vi "Graph mit Bemerkung.vi"(0 "Context (Eingang)":refnum<class "Context.lvclass">, 1 "Table Configuration":T4={"Table Settings"={"Number of Columns"=1, "Width (%)"=100.0, "Relative Column Widths (%)"=[100.0], "Horizontal Align"=0, "Header Rows"=0}, "Cell Defaults"={"Background Color"=16777215, "Horizontal Align"=0, "Vertical Align"=1, "Minimum Height"=0.0, "Fixed Height"=0.0, "Padding"={"Left"=0.0, "Top"=0.0, "Right"=0.0, "Bottom"=0.0}}, "Borders"={"Left"={"Enabled"=FALSE, "Width"=1.0, "Color"=0}, "Top"={"Enabled"=FALSE, "Width"=1.0, "Color"=0}, "Right"={"Enabled"=FALSE, "Width"=1.0, "Color"=0}, "Bottom"={"Enabled"=FALSE, "Width"=1.0, "Color"=0}, "Middle Horizontal"={"Enabled"=FALSE, "Width"=0.5, "Color"=0}, "Middle Vertical"={"Enabled"=FALSE, "Width"=0.5, "Color"=0}}} {"Cell Defaults"."Vertical Align" items=["Bottom", "Middle", "Top"]; "Cell Defaults"."Horizontal Align" items=["Center", "Justified", "JustifiedAll", "Left", "Right"]; "Table Settings"."Horizontal Align" items=["Center"=0, "Left"=3, "Right"=4]}, 2 "Cell Configuration":T1={"Cell Defaults"={"Background Color"=16777215, "Horizontal Align"=0, "Vertical Align"=1, "Minimum Height"=0.0, "Fixed Height"=0.0, "Padding"={"Left"=0.0, "Top"=0.0, "Right"=0.0, "Bottom"=0.0}}, "Borders"={"Left"={"Enabled"=FALSE, "Width"=1.0, "Color"=0}, "Top"={"Enabled"=FALSE, "Width"=1.0, "Color"=0}, "Right"={"Enabled"=FALSE, "Width"=1.0, "Color"=0}, "Bottom"={"Enabled"=FALSE, "Width"=1.0, "Color"=0}}, "Column Span"=0} {"Cell Defaults"."Vertical Align" items=["Bottom", "Middle", "Top"]; "Cell Defaults"."Horizontal Align" items=["Center", "Justified", "JustifiedAll", "Left", "Right"]}, 5 "Graph":T6={"GraphCtl Refnum"=refnum, "Wrap Text (F:No)"=FALSE, "Hide Grid (F:No)"=FALSE, "Scale (100%)"=100.0, "Align (Left)"=0, "PositionBemerkung"=enum."before", "PageBreak"=enum."before"} {"Align (Left)" items=["Center", "Justified", "Justified All", "Left", "Right"]}, 7 "Bemerkung Index (Eingang)":i32, 11 "Fehler (Eingang, kein Fehler)":errorcluster, 12 "Bemerkungen":T10[](array[typedef]) {"Align (Left)" items=["Center", "Justified", "Justified All", "Left", "Right"]}) -> (4 "Context (Ausgang)":refnum<class "Context.lvclass">, 8 "Bemerkung Index (Ausgang)":i32, 15 "Fehler (Ausgang)":errorcluster)   [LabVIEW 2020, in "PDF Interface.lvlib" / "PDF Interface Helper.lvlib"]
uses:
  PDF Interface Helper.lvlib
  PDFBemerkung.ctl
  <vilib>/Simplicity AI/SAI_PDF_API/Classes/Context/Controls/SAI_PDF_Text Align.ctl
  <vilib>/Simplicity AI/SAI_PDF_API/Classes/Context/Controls/SAI_PDF_Font.ctl
  <vilib>/Simplicity AI/SAI_PDF_API/Classes/Context/Controls/SAI_PDF_Font Encoding.ctl
  <vilib>/Simplicity AI/SAI_PDF_API/Classes/Context/Context.lvclass
  PDFGraph.ctl
  PDFCommentPosition.ctl
  PDFPageBreak.ctl
  <vilib>/Simplicity AI/SAI_PDF_API/Classes/Table Builder/Controls/SAI_PDF_Table Configuration.ctl
  <vilib>/Simplicity AI/SAI_PDF_API/Classes/Table Builder/Controls/SAI_PDF_Table Horizontal Align.ctl
  <vilib>/Simplicity AI/SAI_PDF_API/Classes/Table Builder/Controls/SAI_PDF_Default Cell Format.ctl
  <vilib>/Simplicity AI/SAI_PDF_API/Classes/Table Builder/Controls/SAI_PDF_BorderLine.ctl
  <vilib>/Simplicity AI/SAI_PDF_API/Classes/Table Builder/Controls/SAI_PDF_Cell Configuration.ctl
  <vilib>/Simplicity AI/SAI_PDF_API/Classes/Table Builder/Table Builder.lvclass
panel:
  # "(Cp1252)"
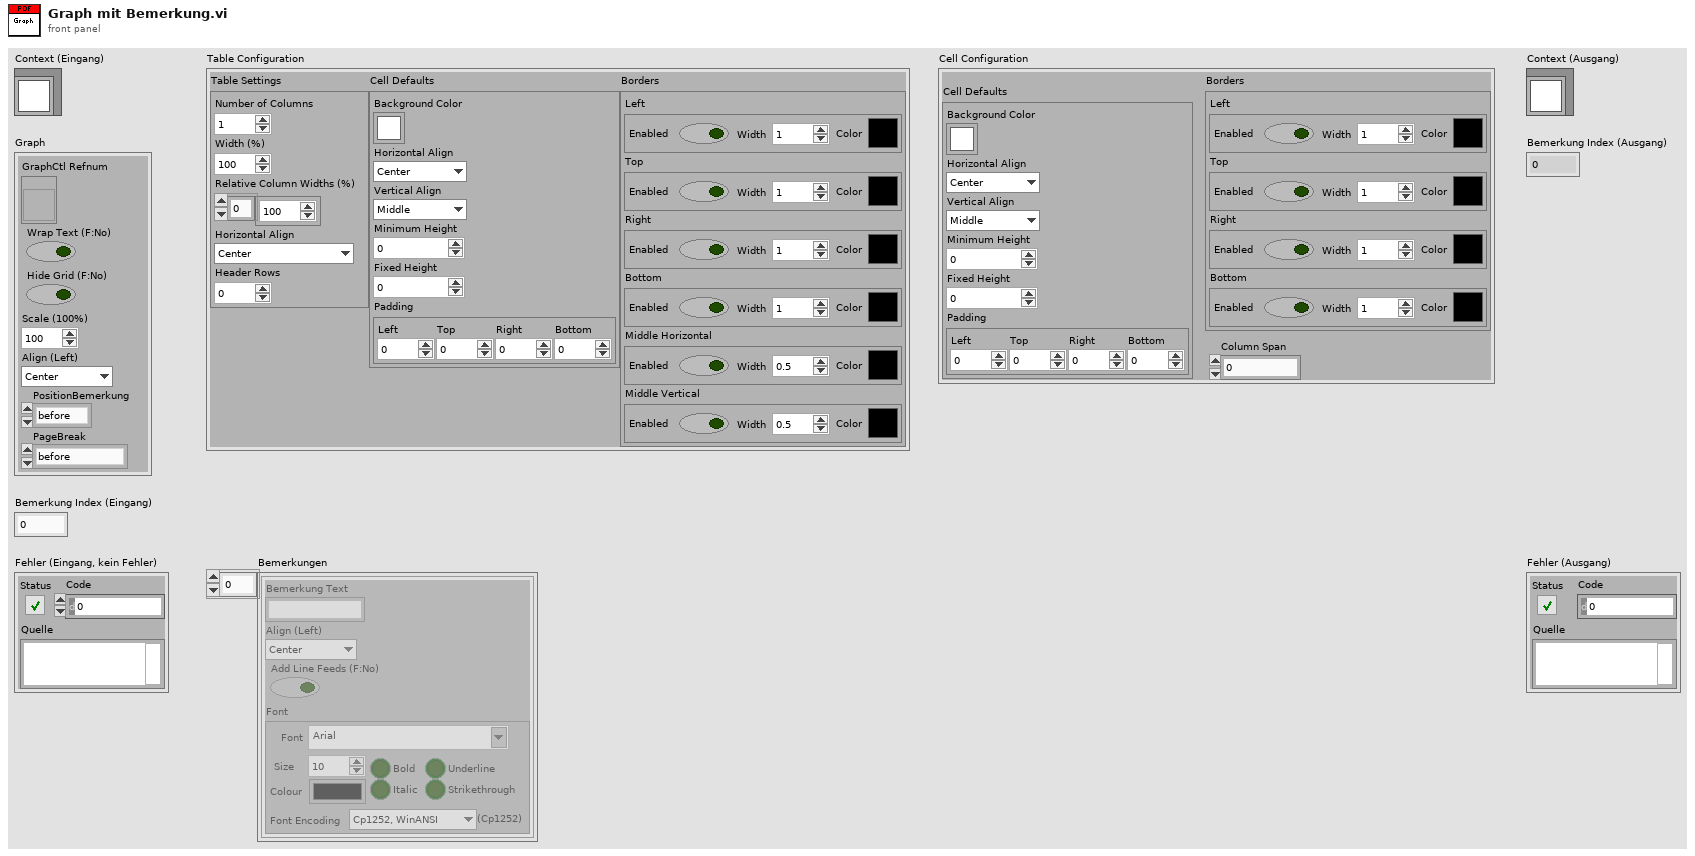
[diagram p1: front panel]
types:
  T1 = typedef "SAI_PDF_Toolkit.lvlib/Table Builder.lvclass/SAI_PDF_Cell Configuration.ctl" = cluster{"Cell Defaults":T2, "Borders":cluster{"Left":T3, "Top":T3, "Right":T3, "Bottom":T3}, "Column Span":i32}
  T2 = typedef "SAI_PDF_Toolkit.lvlib/Table Builder.lvclass/SAI_PDF_Default Cell Format.ctl" = cluster{"Background Color":u32, "Horizontal Align":i32, "Vertical Align":i32, "Minimum Height":sgl, "Fixed Height":sgl, "Padding":cluster{"Left":sgl, "Top":sgl, "Right":sgl, "Bottom":sgl}}
  T3 = typedef "SAI_PDF_Toolkit.lvlib/Table Builder.lvclass/SAI_PDF_BorderLine.ctl" = cluster{"Enabled":bool, "Width":sgl, "Color":u32}
  T4 = typedef "SAI_PDF_Toolkit.lvlib/Table Builder.lvclass/SAI_PDF_Table Configuration.ctl" = cluster{"Table Settings":cluster{"Number of Columns":i32, "Width (%)":sgl, "Relative Column Widths (%)":sgl[], "Horizontal Align":T5, "Header Rows":i32}, "Cell Defaults":T2, "Borders":cluster{"Left":T3, "Top":T3, "Right":T3, "Bottom":T3, "Middle Horizontal":T3, "Middle Vertical":T3}}
  T5 = typedef "SAI_PDF_Toolkit.lvlib/Table Builder.lvclass/SAI_PDF_Table Horizontal Align.ctl" = i32
  T6 = typedef "PDF Interface.lvlib/PDF Interface Helper.lvlib/PDFGraph.ctl" = cluster{"GraphCtl Refnum":refnum<vi>, "Wrap Text (F:No)":bool, "Hide Grid (F:No)":bool, "Scale (100%)":sgl, "Align (Left)":T7, "PositionBemerkung":T8, "PageBreak":T9}
  T7 = typedef "SAI_PDF_Toolkit.lvlib/Context.lvclass/SAI_PDF_Text Align.ctl" = i32
  T8 = typedef "PDF Interface.lvlib/PDF Interface Helper.lvlib/PDFCommentPosition.ctl" = enum16{"before", "after"}
  T9 = typedef "PDF Interface.lvlib/PDF Interface Helper.lvlib/PDFPageBreak.ctl" = enum16{"none", "before", "after", "after comment"}
  T10 = typedef "PDF Interface.lvlib/PDF Interface Helper.lvlib/PDFBemerkung.ctl" = cluster{"Bemerkung Text":string, "Align (Left)":T7, "Add Line Feeds (F:No)":bool, "Font":T11}
  T11 = typedef "SAI_PDF_Toolkit.lvlib/Context.lvclass/SAI_PDF_Font.ctl" = cluster{"Font":string, "Size":i32, "Colour":u32, "Bold":bool, "Italic":bool, "Underline":bool, "Strikethrough":bool, "Font Encoding":T12}
  T12 = typedef "SAI_PDF_Toolkit.lvlib/Context.lvclass/SAI_PDF_Font Encoding.ctl" = enum16{"Cp1252, WinANSI", "IdentityH", "IdentityV", "Cp1250", "Cp1257", "MacRoman"}
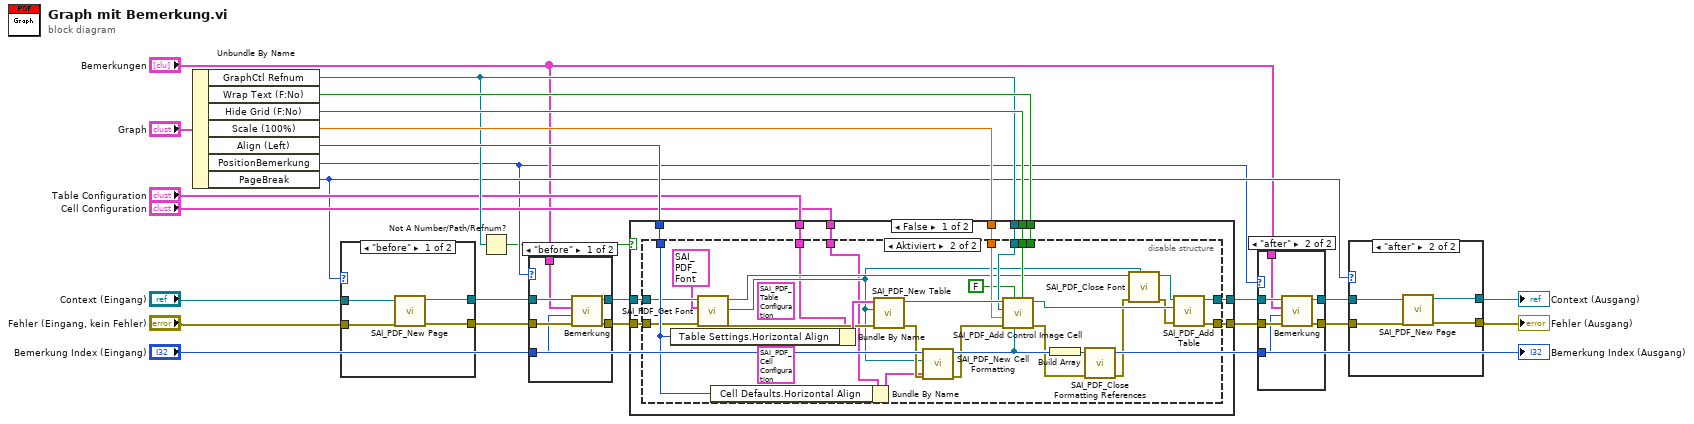
[diagram p0: block diagram]
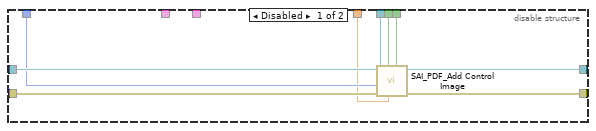
[diagram p2: hidden frame]
diagram:
  n1 = Unbundle By Name("Graph") -> ("GraphCtl Refnum"=w19:refnum<vi>, "Wrap Text (F:No)"=w23:bool, "Hide Grid (F:No)"=w22:bool, "Scale (100%)"=w21:sgl, "Align (Left)"=w20:T7, "PositionBemerkung"=w6:T8, "PageBreak"=w8:T9)
  n2 = case shown="\"before\"" w8 {
    tunnel: "Context (Eingang)" -> [w29 w31]
    tunnel: [w28 w31] -> w16
    tunnel: "Fehler (Eingang, kein Fehler)" -> [w27 w30]
    tunnel: [w26 w30] -> w15
    frame "before" {
      n3 = call <vilib>:"SAI_PDF_New Page.vi"("error in"=w27, "Context In"=w29) -> ("error out"=w26:errorcluster, "Context Out"=w28:refnum<class "Context.lvclass">)  [unwired: 8 in]
    }
    frame "after", Default {
    }
  }
  n4 = Not A Number/Path/Refnum?(number/path/refnum=w19) -> (NaN/Path/Refnum?=w1:bool)
  n5 = case shown="\"before\"" w6 {
    tunnel: w16 -> [w37 w39]
    tunnel: [w36 w39] -> w3
    tunnel: w15 -> [w35 w38]
    tunnel: [w34 w38] -> w2
    tunnel: "Bemerkung Index (Eingang)" -> [w33 _]
    tunnel: "Bemerkungen" -> [w32 _]
    frame "before" {
      n6 = call "Bemerkung.vi"("Fehler (Eingang, kein Fehler)"=w35, "Index"=w33, "Bemerkung"=w32, "Context (Eingang)"=w37) -> ("Fehler (Ausgang)"=w34:errorcluster, "Context (Ausgang)"=w36:refnum<class "Context.lvclass">)  [unwired: 6 in]
    }
    frame "after", Default {
    }
  }
  n7 = case shown="False" w1 {
    tunnel: [w50 w88] -> w5
    tunnel: [w49 w87] -> w4
    tunnel: w19 -> [w48 _]
    tunnel: w23 -> [w47 _]
    tunnel: w22 -> [w46 _]
    tunnel: w20 -> [w45 _]
    tunnel: w21 -> [w44 _]
    tunnel: "Table Configuration" -> [w43 _]
    tunnel: "Cell Configuration" -> [w42 _]
    tunnel: w3 -> [w41 w88]
    tunnel: w2 -> [w40 w87]
    frame False {
      n8 = disable-structure shown="Aktiviert" {
        disable-tunnel: w41 -> [w59 w71]
        disable-tunnel: w40 -> [w58 w70]
        disable-tunnel: [w57 w78] -> w50
        disable-tunnel: [w56 w79] -> w49
        disable-tunnel: w48 -> [w55 w76]
        disable-tunnel: w47 -> [w54 _]
        disable-tunnel: w46 -> [w53 w77]
        disable-tunnel: w45 -> [w52 w72]
        disable-tunnel: w44 -> [w51 w75]
        disable-tunnel: w43 -> [_ w61]
        disable-tunnel: w42 -> [_ w60]
        frame Disabled {
          n9 = call <vilib>:"SAI_PDF_Add Control Image.vi"("Wrap Text (F:No)"=w54, "Scale (100%)"=w51, "Hide Grid (F:No)"=w53, "error in (no error)"=w58, "Align (Left)"=w52, "Ctl Refnum"=w55, "Context In"=w59) -> ("error out"=w56:errorcluster, "Context Out"=w57:refnum<class "Context.lvclass">)  [unwired: 3 in]
        }
        frame Enabled {
          (unwired) T1 {"Cell Defaults"={"Background Color"=16777215, "Horizontal Align"=0, "Vertical Align"=1, "Minimum Height"=0.0, "Fixed Height"=0.0, "Padding"={"Left"=2.0, "Top"=2.0, "Right"=2.0, "Bottom"=3.0}}, "Borders"={"Left"={"Enabled"=TRUE, "Width"=1.0, "Color"=0}, "Top"={"Enabled"=TRUE, "Width"=1.0, "Color"=0}, "Right"={"Enabled"=TRUE, "Width"=1.0, "Color"=0}, "Bottom"={"Enabled"=TRUE, "Width"=1.0, "Color"=0}}, "Column Span"=0} ("Cell Configuration")
          (unwired) T4 {"Table Settings"={"Number of Columns"=1, "Width (%)"=100.0, "Relative Column Widths (%)"=[100.0], "Horizontal Align"=0, "Header Rows"=0}, "Cell Defaults"={"Background Color"=16777215, "Horizontal Align"=0, "Vertical Align"=1, "Minimum Height"=0.0, "Fixed Height"=0.0, "Padding"={"Left"=2.0, "Top"=2.0, "Right"=2.0, "Bottom"=3.0}}, "Borders"={"Left"={"Enabled"=TRUE, "Width"=1.0, "Color"=0}, "Top"={"Enabled"=TRUE, "Width"=1.0, "Color"=0}, "Right"={"Enabled"=TRUE, "Width"=1.0, "Color"=0}, "Bottom"={"Enabled"=TRUE, "Width"=1.0, "Color"=0}, "Middle Horizontal"={"Enabled"=TRUE, "Width"=0.5, "Color"=0}, "Middle Vertical"={"Enabled"=TRUE, "Width"=0.5, "Color"=0}}} ("Table Configuration")
          n10 = Bundle By Name(cluster=w61, "Table Settings.Horizontal Align"=w72) -> (w74:T4)
          n11 = call <vilib>:"SAI_PDF_Get Font.vi"("error in"=w70, "Font"=T11 {"Font"="Arial", "Size"=10, "Colour"=0, "Bold"=FALSE, "Italic"=FALSE, "Underline"=FALSE, "Strikethrough"=FALSE, "Font Encoding"=enum."Cp1252, WinANSI"}, "Context In"=w71) -> ("error out"=w69:errorcluster, "Font"=w63:refnum<class "Font.lvclass">, "Context Out"=w68:refnum<class "Context.lvclass">)  [unwired: 6 out]
          n12 = Bundle By Name(cluster=w60, "Cell Defaults.Horizontal Align"=w72) -> (w73:T1)
          n13 = call <vilib>:"SAI_PDF_New Table.vi"("error in"=w69, "Font In"=w63, "Table Configuration"=w74) -> ("error out"=w81:errorcluster, "Table Builder"=w86:refnum<class "Table Builder.lvclass">)  [unwired: 7 out]
          n14 = call <vilib>:"SAI_PDF_New Cell Formatting.vi"("error in"=w81, "Font In"=w63, "Cell Configuration"=w73) -> ("error out"=w82:errorcluster, "Cell Formatting"=w83:refnum<class "Formatting.lvclass">)  [unwired: 7 out]
          n15 = call <vilib>:"SAI_PDF_Add Control Image Cell.vi"("Hide Grid (F:No)"=w77, "Formatting In"=w83, "Autoscale? (T)"=FALSE, "error in"=w82, "Image Scale (%)"=w75, "Ctl Refnum In"=w76, "Table Builder In"=w86) -> ("error out"=w80:errorcluster, "Table Builder Out"=w85:refnum<class "Table Builder.lvclass">)  [unwired: 3 in]
          n16 = Build Array(w83) -> (w84:refnum<class "Formatting.lvclass">[])
          n17 = call <vilib>:"SAI_PDF_Close Formatting References.vi"("error in"=w80, "Formatting Refs"=w84) -> ("error out"=w66:errorcluster)  [unwired: 9 out]
          n18 = call <vilib>:"SAI_PDF_Close Font.vi"("Font"=w63, "error in"=w66, "Context In"=w68) -> ("error out"=w65:errorcluster, "Context Out"=w67:refnum<class "Context.lvclass">)  [unwired: 7 out]
          n19 = call <vilib>:"SAI_PDF_Add Table.vi"("error in"=w65, "Table Builder In"=w85, "Context In"=w67) -> ("error out"=w79:errorcluster, "Context Out"=w78:refnum<class "Context.lvclass">)  [unwired: 7 out]
        }
      }
    }
    frame True {
    }
  }
  n20 = case shown="\"after\"" w6 {
    tunnel: [w90 w96] -> w12
    tunnel: [w89 w95] -> w9
    tunnel: w5 -> [w90 w94]
    tunnel: w4 -> [w89 w93]
    tunnel: "Bemerkungen" -> [_ w92]
    tunnel: "Bemerkung Index (Eingang)" -> [_ w91]
    frame "before", Default {
    }
    frame "after" {
      n21 = call "Bemerkung.vi"("Fehler (Eingang, kein Fehler)"=w93, "Index"=w91, "Bemerkung"=w92, "Context (Eingang)"=w94) -> ("Fehler (Ausgang)"=w95:errorcluster, "Context (Ausgang)"=w96:refnum<class "Context.lvclass">)  [unwired: 6 in]
    }
  }
  n22 = case shown="\"after\"" w8 {
    tunnel: w12 -> [w98 w102]
    tunnel: [w98 w101] -> w11
    tunnel: w9 -> [w97 w100]
    tunnel: [w97 w99] -> w10
    frame "before", Default {
    }
    frame "after" {
      n23 = call <vilib>:"SAI_PDF_New Page.vi"("error in"=w100, "Context In"=w102) -> ("error out"=w99:errorcluster, "Context Out"=w101:refnum<class "Context.lvclass">)  [unwired: 8 in]
    }
  }
  "Fehler (Ausgang)" <- w10
  "Context (Ausgang)" <- w11
  "Bemerkung Index (Ausgang)" <- "Bemerkung Index (Eingang)"
